vi "Write U64.vi"(8 "error in":errorcluster, 9 "value in":u64, 10 "register name":string, 11 "session in":u32) -> (0 "error out":errorcluster, 3 "session out":u32)   [LabVIEW 2018, in "Scalar IO Operations.lvlib"]
uses:
  Scalar IO Operations.lvlib
  NiFpga.dll
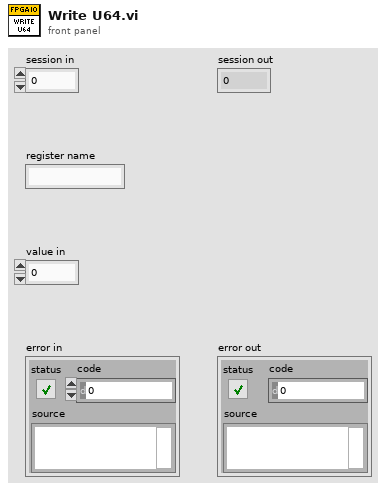
[diagram p1: front panel]
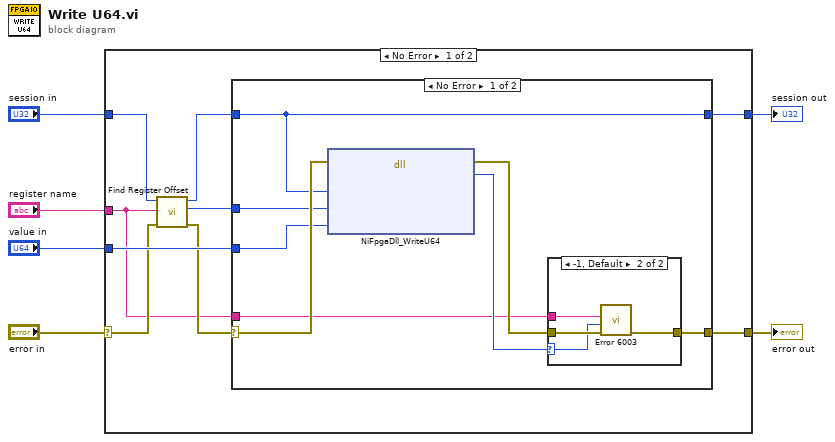
[diagram p0: block diagram]
diagram:
  n1 = case shown="No Error" "error in" {
    selector: "error in" -> [w9 w31]
    tunnel: "session in" -> [w12 w32]
    tunnel: [w15 w31] -> w5
    tunnel: [w14 w32] -> w4
    tunnel: "value in" -> [w13 _]
    tunnel: "register name" -> [w7 _]
    frame No Error {
      n2 = call "Find Register Offset.vi"("error in (no error)"=w9, "register name"=w7, "session in"=w12) -> ("error out"=w8:errorcluster, "resource offset"=w10:u32, "session out"=w11:u32)  [unwired: 6 in]
      n3 = case shown="No Error" w8 {
        selector: w8 -> [w23 w30]
        tunnel: w11 -> [w22 w29]
        tunnel: [w16 w30] -> w15
        tunnel: [w22 w29] -> w14
        tunnel: w13 -> [w21 _]
        tunnel: w10 -> [w20 _]
        tunnel: w7 -> [w17 _]
        frame No Error {
          n4 = dll-call lib="NiFpga.*" fn="NiFpgaDll_WriteU64"(error in=w23, "session"=w22, "offset"=w20, "value"=w21) -> (error out=w19:errorcluster, "status"=w18:i32)  [unwired: 5 in, 1 out]
          n5 = case shown="-1, Default" w18 {
            selector: w18 -> [_ w25]
            tunnel: w19 -> [w24 w28]
            tunnel: [w24 w27] -> w16
            tunnel: w17 -> [_ w26]
            frame 0 {
            }
            frame -1, Default {
              n6 = call "Error 6003.vi"("error in (no error)"=w28, "rio status code"=w25, "register name"=w26) -> ("error out"=w27:errorcluster)  [unwired: 8 in]
            }
          }
        }
        frame Error {
        }
      }
    }
    frame Error {
    }
  }
  "error out" <- w5
  "session out" <- w4
